vi "GetText.vi"(8 "error in":errorcluster, 11 "tag select module editor node in":refnum<class "tag select module editor node.lvclass">) -> (0 "error out":errorcluster, 1 "additional text":string, 2 "text":string, 3 "tag select module editor node out":refnum<class "tag select module editor node.lvclass">, 4 "glyph":string)   [LabVIEW 2014, in "tag select module editor node.lvclass"]
uses:
  tag select module editor node.lvclass
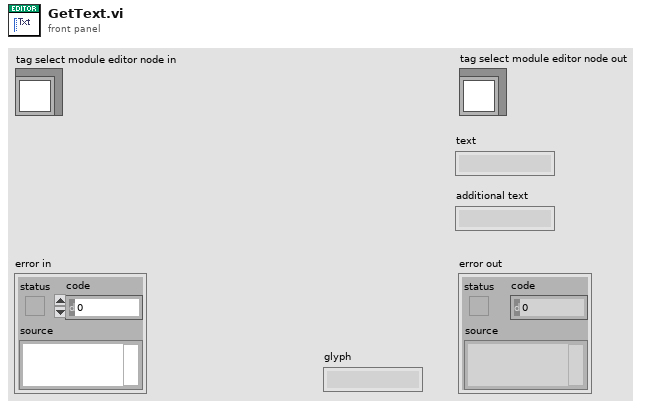
[diagram p1: front panel]
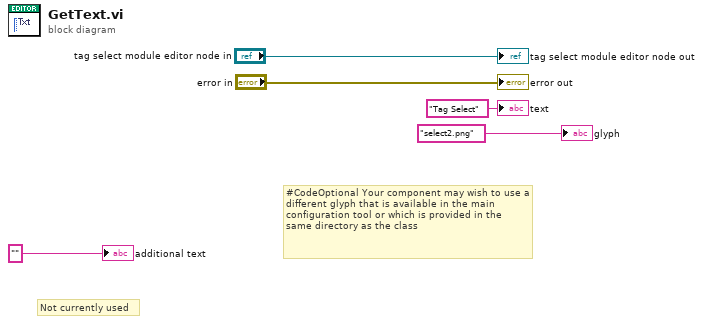
[diagram p0: block diagram]
diagram:
  # "Not currently used"
  # "#CodeOptional Your component may wish to use a different glyph that is available in the main configuration tool or which is provided in the same directory as the class"
  "error out" <- "error in"
  "tag select module editor node out" <- "tag select module editor node in"
  "text" <- "Tag Select" ("text")
  "additional text" <- "" ("additional text")
  "glyph" <- "select2.png" ("glyph")
